vi "Ready Busy Status.vi"(8 "error in (no error)":errorcluster, 11 "XY Stage Controller in":refnum<class "XY Stage Controller.lvclass">) -> (0 "error out":errorcluster, 2 "Busy":bool, 3 "XY Stage Controller out":refnum<class "XY Stage Controller.lvclass">)   [LabVIEW 2022 SP3, in "XY Stage Controller.lvclass"]
uses:
  XY Stage Controller.lvclass
  XY Stage Controller.lvclass/XY Stage Controller.ctl
  Process Framework/Process State Data/Process State Data.lvclass
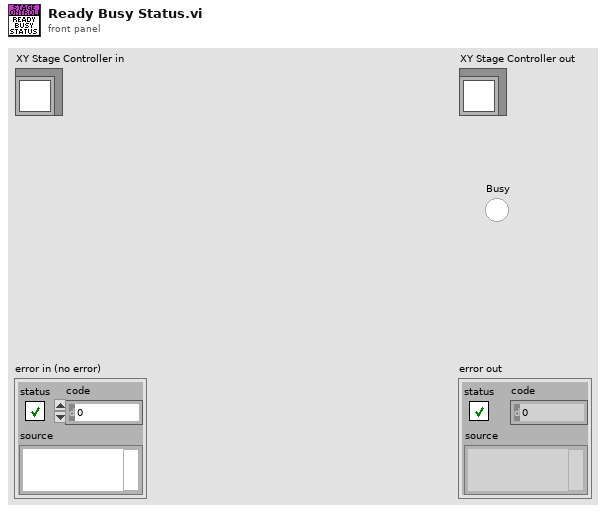
[diagram p1: front panel]
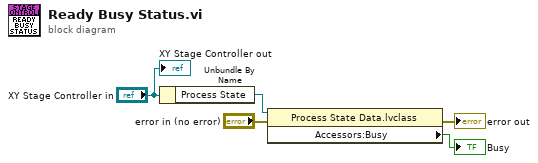
[diagram p0: block diagram]
diagram:
  n1 = Unbundle By Name("XY Stage Controller in") -> ("Process State"=w4:refnum<data-value>)
  n2 = property class="Process State Data.lvclass"(reference=w4, error in="error in (no error)") -> (error out=→"error out":errorcluster, "Accessors:Busy"=→"Busy":bool)  [unwired: 1 out]
  "XY Stage Controller out" <- "XY Stage Controller in"
